vi "Run Bfr Rx - Timed RT.vi"(7 "Process in":refnum<class "Process.lvclass">, 8 "error in (no error)":errorcluster, 11 "Rx Loop Data in":T1 {"Buffer Resources"."Data Buffer" format="%016x"; "Buffer Option Support"."Cached Buffer"."Cache Buffer" format="%016x"}) -> (3 "Rx Loop Data out":T1 {"Buffer Resources"."Data Buffer" format="%016x"; "Buffer Option Support"."Cached Buffer"."Cache Buffer" format="%016x"})   [LabVIEW 2016, in "UDP-Custom-Device Engine.lvlib"]
uses:
  UDP-Custom-Device Engine.lvlib
  <vilib>/NI/NIVS Inline Async API/_VS Inline Async API/Process/Process.lvclass
  Types/Engine - Buffered Rx Loop Data.ctl
  Types/Engine - General Resources.ctl
  <vilib>/NI Veristand/VeriStand Data/Typedefs/Typedefs.Data Types.ctl
  Shared/Types/Shared - Duplex Settings.ctl
  Shared/Types/Shared - Header Details.ctl
  Types/Engine - Buffer Resources.ctl
  Shared/Types/Shared - Pointer Encoding.ctl
  Types/Engine - Rx Runtime Resources.ctl
  Types/Engine - Execution Config.ctl
  Shared/Types/Shared - Thread Management.ctl
  Types/Engine - Rx New Data Options Support.ctl
  Shared/Types/Shared - New Data Options.ctl
  Types/Engine - Buffered Rx Buffer Option Support.ctl
  Shared/Types/Shared - Receive Buffer Options.ctl
  Types/Engine - Buffered Rx Circular Buffer.ctl
  Types/Engine - Buffered Rx Cached Buffer.ctl
  Types/Engine - Buffered Rx Channel Refs.ctl
  <vilib>/NI/NIVS Inline Async API/_Data Access Engine/Data Access Engine/Types/Write.DVR.ctl
  <vilib>/NI/NIVS Inline Async API/_Data Access Engine/Access Type Classes/Write/Write.lvclass
  <vilib>/NI/NIVS Inline Async API/_Data Access Engine/Data Access Engine/Types/Read.DVR.ctl
  <vilib>/NI/NIVS Inline Async API/_Data Access Engine/Access Type Classes/Read/Read.lvclass
  Types/Engine - Debug Resources.ctl
  <vilib>/Platform/TimedLoop/XDataNode/timing_clust.ctl
  <vilib>/Platform/TimedLoop/XDataNode/nitl_modes.ctl
  <vilib>/Platform/TimedLoop/XDataNode/wakeup.ctl
  <vilib>/NI/NIVS Inline Async API/_Data Access Engine/Access Type Classes/Read/Read.lvclass/Read.ctl
  <vilib>/NI/NIVS Inline Async API/_Data Access Engine/Access Type Classes/Write/Write.lvclass/Write.ctl
  <vilib>/NI/NIVS Inline Async API/_VS Inline Async API/Process/Process.lvclass/Process.ctl
  <vilib>/NI Veristand/VeriStand Data/Type Conversion/Type Conversion.To Double (U64).vi
  <vilib>/NI/NIVS Inline Async API/_Data Access Engine/Data Access Engine/Methods/Write.Data.vi
  <vilib>/NI/NIVS Inline Async API/_Data Access Engine/Data Access Engine/Methods/Read.Data.vi
  <vilib>/NI Veristand/VeriStand Data/Pointer Operations/Pointer.Write.vi
  <vilib>/NI Veristand/VeriStand Data/Pointer Operations/Pointer.Write (1D U8).vi
  Run Bfr Rx - Handle Offset.vi
  Run Bfr Rx - Handle Rollover.vi
  Circular Buffer and Size/Run Bfr Rx - Sized Detect Rollover.vi
  Circular Buffer and Size/Run Bfr Rx - Sized Handle Rollover.vi
  Circular Buffer and Size/Run Bfr Rx - Sized Write Buffer.vi
  <vilib>/NI/NIVS Inline Async API/_Data Access Engine/Access Type Classes/Write/Write.ProcessData.vi
  <vilib>/NI Veristand/VeriStand Data/Type Conversion/Type Conversion.To Double (U16).vi
  <vilib>/NI/NIVS Inline Async API/_VS Inline Async API/Error Handling Process/SubVIs/Error.ConvertArray.vi
  <vilib>/NI/NIVS Inline Async API/_Data Access Engine/Access Type Classes/Read/Read.ProcessData.vi
  <vilib>/NI Veristand/VeriStand Data/Pointer Operations/Pointer.Write (I32).vi
  <vilib>/platform/TimedLoop/XDataNode/XDataNode.xnode
  <vilib>/Platform/TimedLoop/XDataNode/XDNodeRunTimeDep.lvlib
  <vilib>/NI Veristand/VeriStand Data/VeriStand Data.lvlib
  <vilib>/NI/NIVS Inline Async API/_Data Access Engine/Data Access Engine/Data Access Engine.lvclass
  Shared/UDP-Custom-Device Shared.lvlib
panel:
  out "dataBuffer":u64 format="%016x"
  out "dataLength":u64
  out "newData":string
  # "BUFFERED RECEIVE\n- TIMED\n- REALTIME ONLY"
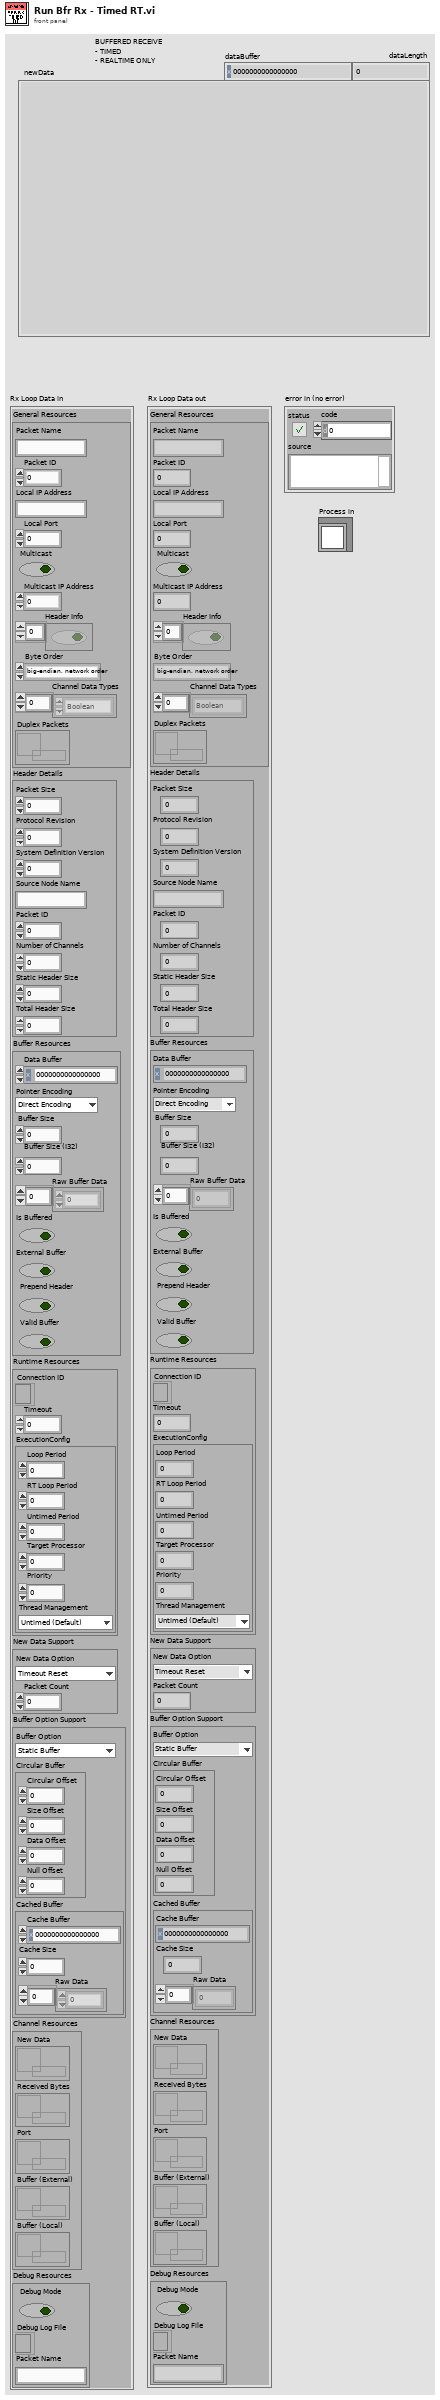
[diagram p1: front panel]
types:
  T1 = typedef "UDP-Custom-Device Engine.lvlib/Engine - Buffered Rx Loop Data.ctl" = cluster{"General Resources":T2, "Header Details":T4, "Buffer Resources":T5, "Runtime Resources":T7, "New Data Support":T10, "Buffer Option Support":T12, "Channel Resources":T16, "Debug Resources":T19}
  T2 = typedef "UDP-Custom-Device Engine.lvlib/Engine - General Resources.ctl" = cluster{"Packet Name":string, "Packet ID":i32, "Local IP Address":string, "Local Port":i32, "Multicast":bool, "Multicast IP Address":u32, "Header Info":bool[], "Byte Order":enum16{"big-endian, network order", "native, host order", "little-endian"}, "Channel Data Types":T3[], "Duplex Packets":refnum<data-value>}
  T3 = typedef "VeriStand Data.lvlib/Typedefs.Data Types.ctl" = enum16{"Boolean", "Single", "Double", "I8", "I16", "I32", "I64", "U8", "U16", "U32", "U64"}
  T4 = typedef "UDP-Custom-Device Shared.lvlib/Shared - Header Details.ctl" = cluster{"Packet Size":u16, "Protocol Revision":u8, "System Definition Version":u64, "Source Node Name":string, "Packet ID":u32, "Number of Channels":u32, "Static Header Size":u16, "Total Header Size":u16}
  T5 = typedef "UDP-Custom-Device Engine.lvlib/Engine - Buffer Resources.ctl" = cluster{"Data Buffer":u64, "Pointer Encoding":T6, "Buffer Size":u64, "Buffer Size (I32)":i32, "Raw Buffer Data":u8[], "Is Buffered":bool, "External Buffer":bool, "Prepend Header":bool, "Valid Buffer":bool}
  T6 = typedef "UDP-Custom-Device Shared.lvlib/Shared - Pointer Encoding.ctl" = enum16{"Direct Encoding", "Conversion Encoding"}
  T7 = typedef "UDP-Custom-Device Engine.lvlib/Engine - Rx Runtime Resources.ctl" = cluster{"Connection ID":refnum<k16>, "Timeout":i32, "ExecutionConfig":T8}
  T8 = typedef "UDP-Custom-Device Engine.lvlib/Engine - Execution Config.ctl" = cluster{"Loop Period":i64, "RT Loop Period":i64, "Untimed Period":u32, "Target Processor":i32, "Priority":i32, "Thread Management":T9}
  T9 = typedef "UDP-Custom-Device Shared.lvlib/Shared - Thread Management.ctl" = enum16{"Untimed (Default)", "Timed (High Priority)"}
  T10 = typedef "UDP-Custom-Device Engine.lvlib/Engine - Rx New Data Options Support.ctl" = cluster{"New Data Option":T11, "Packet Count":dbl}
  T11 = typedef "UDP-Custom-Device Shared.lvlib/Shared - New Data Options.ctl" = enum16{"Timeout Reset", "Counter"}
  T12 = typedef "UDP-Custom-Device Engine.lvlib/Engine - Buffered Rx Buffer Option Support.ctl" = cluster{"Buffer Option":T13, "Circular Buffer":T14, "Cached Buffer":T15}
  T13 = typedef "UDP-Custom-Device Shared.lvlib/Shared - Receive Buffer Options.ctl" = enum16{"Static Buffer", "Circular Buffer", "Circular Buffer + Size", "Block Cache", "Block Cache + Size"}
  T14 = typedef "UDP-Custom-Device Engine.lvlib/Engine - Buffered Rx Circular Buffer.ctl" = cluster{"Circular Offset":u64, "Size Offset":u64, "Data Offset":u64, "Null Offset":u64}
  T15 = typedef "UDP-Custom-Device Engine.lvlib/Engine - Buffered Rx Cached Buffer.ctl" = cluster{"Cache Buffer":u64, "Cache Size":u64, "Raw Data":u8[]}
  T16 = typedef "UDP-Custom-Device Engine.lvlib/Engine - Buffered Rx Channel Refs.ctl" = cluster{"New Data":T17, "Received Bytes":T17, "Port":T17, "Buffer (External)":T18, "Buffer (Local)":T17}
  T17 = typedef "Data Access Engine.lvlib/Data Access Engine.lvclass/Write.DVR.ctl" = refnum<data-value>
  T18 = typedef "Data Access Engine.lvlib/Data Access Engine.lvclass/Read.DVR.ctl" = refnum<data-value>
  T19 = typedef "UDP-Custom-Device Engine.lvlib/Engine - Debug Resources.ctl" = cluster{"Debug Mode":bool, "Debug Log File":refnum<file>, "Packet Name":string}
  T20 = typedef "XDNodeRunTimeDep.lvlib/timing_clust.ctl" = cluster{"Expected End [f-1]":u64, "Actual End [f-1]":u64, "Finished Late? [f-1]":bool, "Expected End [i-1]":u64, "Actual End [i-1]":u64, "Finished Late? [i-1]":bool, "Expected Start [i]":u64, "Actual Start [i]":u64, "Expected Start [f]":u64, "Actual Start [f]":u64, "Source Name":string, "Structure Name":string, "Period":i64, "Deadline":i64, "Offset":i64, "Start":i64, "Priority":i32, "Timeout":i32, "Mode":T21, "Wakeup Reason":T22, "Error":errorcluster, "Source Type":string, "Secondary Source Type":string, "Global End Time":u64, "Global Start Time":u64, "Frame Duration":u64, "Iteration Duration":u64, "Assigned CPU":i32, "I/O Scan Engine Mode":u32}
  T21 = typedef "XDNodeRunTimeDep.lvlib/nitl_modes.ctl" = enum32{"No Change", "Process missed periods, maintain original phase", "Discard missed periods, maintain original phase", "Process missed periods, ignore original phase", "Discard missed periods, ignore original phase"}
  T22 = typedef "XDNodeRunTimeDep.lvlib/wakeup.ctl" = enum32{"Normal", "Aborted", "Asynchronous wakeup", "Timing source error", "Timed loop error", "Timeout"}
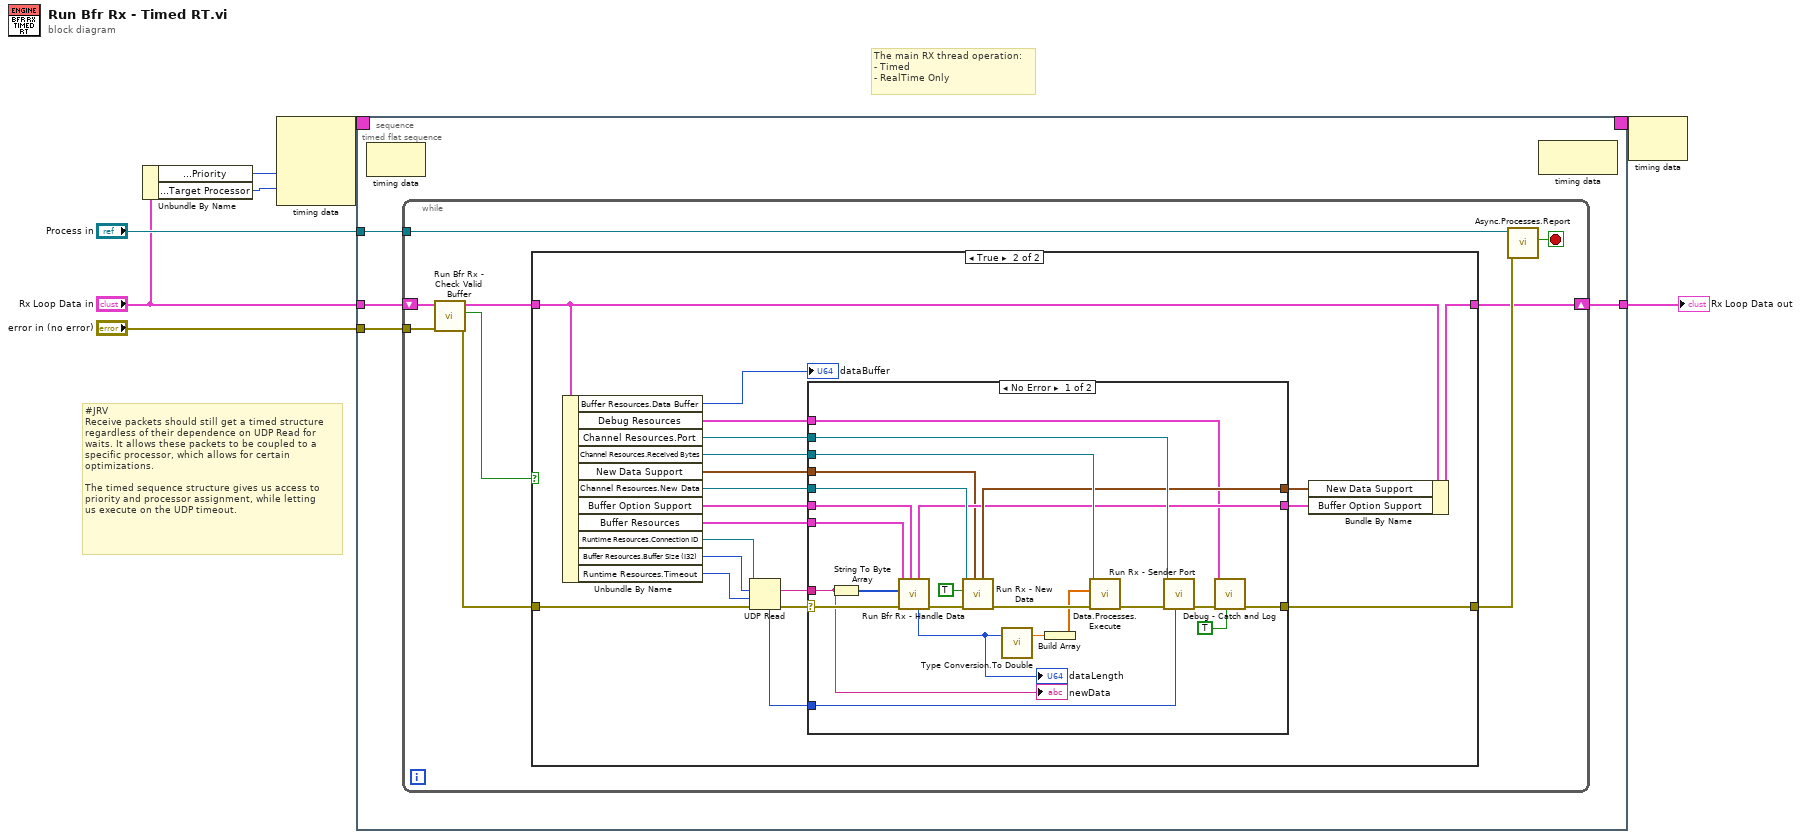
[diagram p0: block diagram]
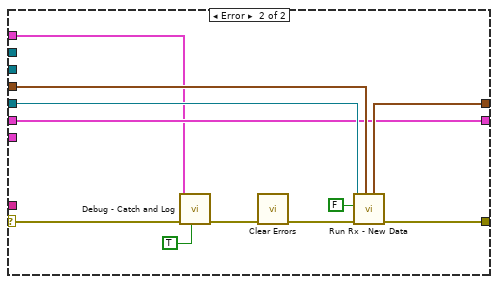
[diagram p3: hidden frame]
diagram:
  # "#JRV\nReceive packets should still get a timed structure\nregardless of their dependence on UDP Read for\nwaits. It allows these packets to be coupled to a\nspecific processor, which allows for certain \noptimizations.\n\nThe timed sequence structure gives us access to\npriority and processor assignment, while letting\nus execute on the UDP timeout."
  # "The main RX thread operation:\n- Timed\n- RealTime Only"
  n1 = Unbundle By Name("Rx Loop Data in") -> ("Runtime Resources.ExecutionConfig.Priority"=w1:i32, "Runtime Resources.ExecutionConfig.Target Processor"=w3:i32)
  n2 = node-c288(w1, w3) -> (w8:T20)  [unwired: 2 in]
  n3 = timed-sequence {
    timing: w8 -> [_]
    timing-out: [_] -> w7
    tunnel: "Process in" -> [w12]
    tunnel: "error in (no error)" -> [w11]
    tunnel: "Rx Loop Data in" -> [w10]
    tunnel: [w9] -> w4
    n4 = timed-flat-sequence {
      tunnel: w12 -> [w16]
      tunnel: w11 -> [w15]
      tunnel: w10 -> [w14]
      tunnel: [w13] -> w9
      n5 = node-c288() -> ()  [unwired: 1 in, 1 out]
      n6 = while {
        tunnel: w15 -> [w19]
        tunnel: w16 -> [w25]
        shift-right: [w22] -> w13
        shift-left: w14 -> [w17]
        stop <- w24 stop-if-true
        n7 = call "Run Bfr Rx - Check Valid Buffer.vi"("error in (no error)"=w19, "Rx Loop Data in"=w17) -> ("error out"=w18:errorcluster, "Allow Rx?"=w20:bool, "Rx Loop Data out"=w21:T1)  [unwired: 7 in]
        n8 = case shown="True" w20 {
          tunnel: w21 -> [w26 w37]
          tunnel: w18 -> [w27 w45]
          tunnel: [w27 w43] -> w23
          tunnel: [w26 w36] -> w22
          frame False {
            # "Invalid buffer. Wait for us to have one that we can use."
          }
          frame True {
            n9 = Unbundle By Name(w37) -> ("Buffer Resources.Data Buffer"=→"dataBuffer":u64, "Debug Resources"=w33:T19, "Channel Resources.Port"=w39:T17, "Channel Resources.Received Bytes"=w40:T17, "New Data Support"=w32:T10, "Channel Resources.New Data"=w41:T17, "Buffer Option Support"=w34:T12, "Buffer Resources"=w31:T5, "Runtime Resources.Connection ID"=w47:refnum<k16>, "Buffer Resources.Buffer Size (I32)"=w29:i32, "Runtime Resources.Timeout"=w46:i32)
            n10 = UDP Read(connection ID=w47, max size (548)=w29, timeout ms (25000)=w46, 8:w45) -> (data out=w44:string, error out=w42:errorcluster, 4:w38:u16)  [unwired: 2 out]
            n11 = case shown="No Error" w42 {
              selector: w42 -> [w59 w73]
              tunnel: w34 -> [w56 w75]
              tunnel: w44 -> [w48 _]
              tunnel: [w52 w78] -> w43
              tunnel: w41 -> [w70 w80]
              tunnel: w40 -> [w68 _]
              tunnel: w39 -> [w64 _]
              tunnel: w38 -> [w62 _]
              tunnel: w32 -> [w51 w77]
              tunnel: [w61 w76] -> w35
              tunnel: [w57 w75] -> w30
              tunnel: w33 -> [w54 w71]
              tunnel: w31 -> [w50 _]
              frame No Error {
                n12 = String To Byte Array(string=w48) -> (unsigned byte array=w60:u8[])
                n13 = call "Run Bfr Rx - Handle Data.vi"("Buffer Option Support in"=w56, "error in (no error)"=w59, "Data"=w60, "Buffer Resources"=w50) -> ("error out"=w58:errorcluster, "Data Size"=w49:u64, "Buffer Option Support out"=w57:T12)  [unwired: 5 in]
                "dataLength" <- w49
                n14 = call "Run Rx - New Data.vi"("New Data Support in"=w51, "error in (no error)"=w58, "New Data"=TRUE, "New Data Ref"=w70) -> ("error out"=w67:errorcluster, "New Data Support out"=w61:T10)  [unwired: 6 in]
                n15 = call-poly <vilib>:"Type Conversion.To Double.vi"("value in"=w49) -> ("value out"=w66:dbl)  [unwired: 2 in]
                n16 = Build Array(w66) -> (w65:dbl[])
                n17 = call-poly <vilib>:"Data.Processes.Execute.vi"("error in (no error)"=w67, "Values"=w65, "Ref"=w68) -> ("error out"=w63:errorcluster)  [unwired: 8 in]
                n18 = call "Run Rx - Sender Port.vi"("Port"=w62, "error in (no error)"=w63, "Port Ref"=w64) -> ("error out"=w53:errorcluster)  [unwired: 8 in]
                n19 = call "Debug - Catch and Log.vi"("Clear Error?"=TRUE, "error in (no error)"=w53, "Debug Resources"=w54) -> ("error out"=w52:errorcluster)  [unwired: 8 in]
                "newData" <- w48
              }
              frame Error {
                n20 = call "Debug - Catch and Log.vi"("Clear Error?"=TRUE, "error in (no error)"=w73, "Debug Resources"=w71) -> ("error out"=w72:errorcluster)  [unwired: 8 in]
                n21 = call <vilib>:"Clear Errors.vi"("error in (no error)"=w72) -> ("error out"=w79:errorcluster)  [unwired: 5 in, 1 out]
                n22 = call "Run Rx - New Data.vi"("New Data Support in"=w77, "error in (no error)"=w79, "New Data"=FALSE, "New Data Ref"=w80) -> ("error out"=w78:errorcluster, "New Data Support out"=w76:T10)  [unwired: 6 in]
              }
            }
            n23 = Bundle By Name(cluster=w37, "New Data Support"=w35, "Buffer Option Support"=w30) -> (w36:T1)
          }
        }
        n24 = call <vilib>:"Async.Processes.Report.vi"("Error"=w23, "Process in"=w25) -> ("Stop"=w24:bool)  [unwired: 8 in, 1 out]
      }
      n25 = node-c288() -> ()  [unwired: 1 in, 1 out]
    }
  }
  "Rx Loop Data out" <- w4
  n26 = node-c288(w7) -> ()  [unwired: 1 out]
